vi "Move Conveyer Belt.vi"(3 "Frisbee States":T1, 4 "Enable Stack":bool, 5 "Suck":bool) -> (1 "move conveyer belt":bool)   [LabVIEW 2012]
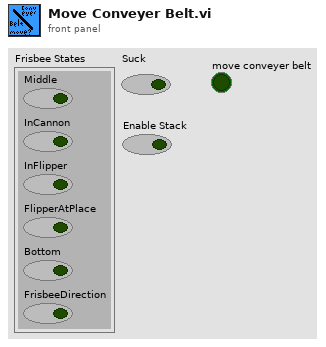
[diagram p1: front panel]
types:
  T1 = cluster{"Middle":bool, "InCannon":bool, "InFlipper":bool, "FlipperAtPlace":bool, "Bottom":bool, "FrisbeeDirection":bool}
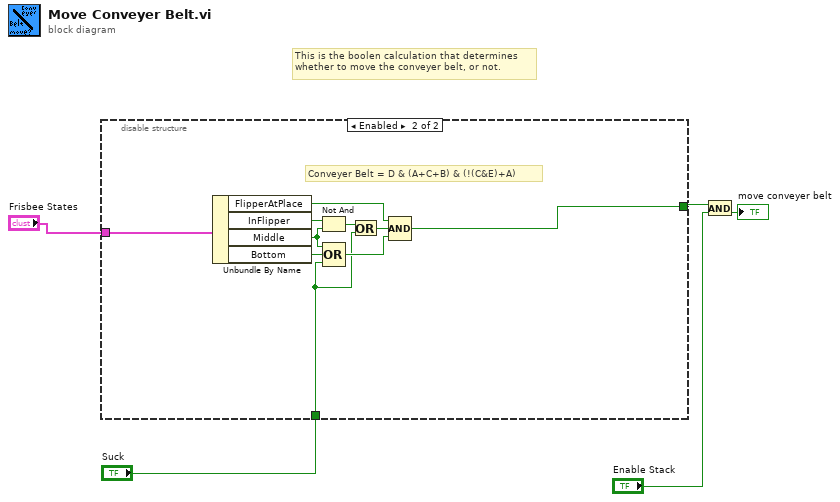
[diagram p0: block diagram]
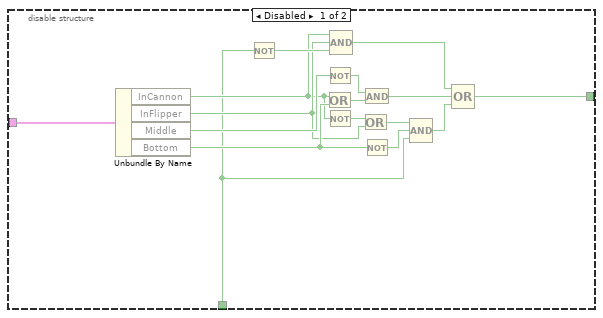
[diagram p2: hidden frame]
diagram:
  # "This is the boolen calculation that determines\nwhether to move the conveyer belt, or not."
  n1 = disable-structure shown="Enabled" {
    disable-tunnel: [w8 w29] -> w2
    disable-tunnel: "Suck" -> [w7 w23]
    disable-tunnel: "Frisbee States" -> [w6 w31]
    frame Disabled {
      n2 = Unbundle By Name(w6) -> ("InCannon"=w10:bool, "InFlipper"=w11:bool, "Middle"=w18:bool, "Bottom"=w15:bool)
      n3 = Not(x=w7) -> (.not. x?=w12:bool)
      n4 = Not(x=w18) -> (.not. x?=w17:bool)
      n5 = Or(x=w10, y=w15) -> (x .or. y?=w16:bool)
      n6 = Not(x=w10) -> (.not. x?=w20:bool)
      n7 = Compound Arithmetic op=AND(w10, w11, w12) -> (w9:bool)
      n8 = Or(x=w20, y=w11) -> (x .or. y?=w19:bool)
      n9 = And(x=w17, y=w16) -> (x .and. y?=w14:bool)
      n10 = Not(x=w15) -> (.not. x?=w21:bool)
      n11 = Compound Arithmetic op=AND(w19, w21, w7) -> (w13:bool)
      n12 = Compound Arithmetic op=OR(w9, w14, w13) -> (w8:bool)
    }
    frame Enabled {
      # "Conveyer Belt = D & (A+C+B) & (!(C&E)+A)"
      n13 = Unbundle By Name(w31) -> ("FlipperAtPlace"=w28:bool, "InFlipper"=w26:bool, "Middle"=w25:bool, "Bottom"=w30:bool)
      n14 = Not And(1:w25, 2:w26) -> (0:w24:bool)
      n15 = Compound Arithmetic op=OR(w25, w30, w23) -> (w27:bool)
      n16 = Or(x=w24, y=w23) -> (x .or. y?=w22:bool)
      n17 = Compound Arithmetic op=AND(w28, w22, w27) -> (w29:bool)
    }
  }
  n18 = And(x=w2, y="Enable Stack") -> (x .and. y?=→"move conveyer belt":bool)
